vi "Get Angle.vi"(5 "register bus":T3={"Speed"="Speed", "Crank Angle"="Crank Angle", "Cycle Angle"="Cycle Angle", "Crank Count"="Crank Count", "Cycle Count"="Cycle Count", "1.25 MHz Counter"="1.25 MHz Counter", "Crank Rollover"="Crank Rollover", "Cycle Rollover"="Cycle Rollover", "shared settings"={"start"=0.0, "stuck limit"=0.0}} {"shared settings"."start" format="%#.15g"}, 6 "settings.<user name>":T5, 7 "input.<user name>":T2, 11 "state data in":T1) -> (3 "state data out":T1)   [LabVIEW 2013, in "Engine Simulation Toolkit.lvlib" / "Digital Pattern Generation.lvlib"]
uses:
  Digital Pattern Generation.lvlib
  Settings.ctl
  APU/Register Bus.ctl
  APU/Shared Settings.ctl
  Input.ctl
  state data.ctl
  <vilib>/rvi/DataTransferAndStorage/Container/Common/niFpgaContainerExecOnDevCompGetState.vi
  <vilib>/rvi/DataTransferAndStorage/Register/Emulation/niFpgaRegisterEmulationFpgaImpl.vi
  <instcachedir>/0/niFpgaRegisterEmulationFpgaImpl_DCF4BC0110594B98B44A971D60CEEC4D.lvgen/niFpgaRegisterEmulationFpgaImpl_DCF4BC0110594B98B44A971D60CEEC4D_006.vi
  <vilib>/rvi/DataTransferAndStorage/Container/Common/niFpgaContainerGetUniqueNameForEmu.vi
  <vilib>/rvi/DataTransferAndStorage/Container/XNode/niFpgaContainer.xnode
  <vilib>/rvi/DataTransferAndStorage/Register/Emulation/niFpgaRegisterEmulationRefIn.vi
  APU/APU.lvlib
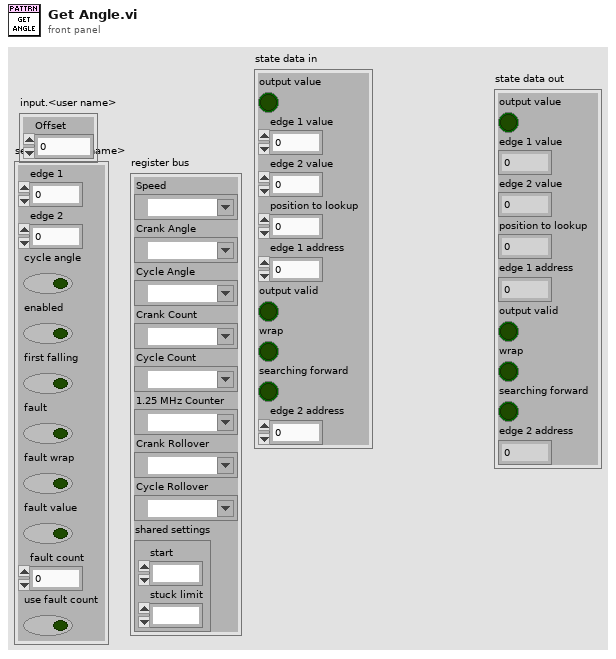
[diagram p1: front panel]
types:
  T1 = typedef "Engine Simulation Toolkit.lvlib/Digital Pattern Generation.lvlib/state data.ctl" = cluster{"output value":bool, "edge 1 value":u16, "edge 2 value":u16, "position to lookup":u16, "edge 1 address":fxp<+,11,11>, "output valid":bool, "wrap":bool, "searching forward":bool, "edge 2 address":fxp<+,11,11>}
  T2 = typedef "Engine Simulation Toolkit.lvlib/Digital Pattern Generation.lvlib/Input.ctl" = cluster{"Offset":i16}
  T3 = typedef "Engine Simulation Toolkit.lvlib/APU.lvlib/Register Bus.ctl" = cluster{"Speed":refnum<k21>, "Crank Angle":refnum<k21>, "Cycle Angle":refnum<k21>, "Crank Count":refnum<k21>, "Cycle Count":refnum<k21>, "1.25 MHz Counter":refnum<k21>, "Crank Rollover":refnum<k21>, "Cycle Rollover":refnum<k21>, "shared settings":T4}
  T4 = typedef "Engine Simulation Toolkit.lvlib/APU.lvlib/Shared Settings.ctl" = cluster{"start":fxp<+,17,17>, "stuck limit":fxp<+,18,18>}
  T5 = typedef "Engine Simulation Toolkit.lvlib/Digital Pattern Generation.lvlib/Settings.ctl" = cluster{"edge 1":u16, "edge 2":u16, "cycle angle":bool, "enabled":bool, "first falling":bool, "fault":bool, "fault wrap":bool, "fault value":bool, "fault count":fxp<+,4,4>, "use fault count":bool}
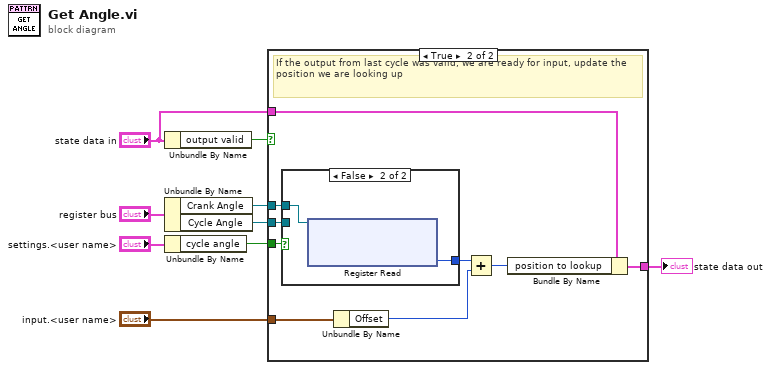
[diagram p0: block diagram]
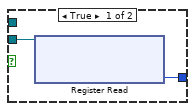
[diagram p3: hidden frame]
diagram:
  n1 = Unbundle By Name("state data in") -> ("output valid"=w1:bool)
  n2 = Unbundle By Name("register bus") -> ("Crank Angle"=w4:refnum<k21>, "Cycle Angle"=w6:refnum<k21>)
  n3 = Unbundle By Name("settings.<user name>") -> ("cycle angle"=w7:bool)
  n4 = case shown="True" w1 {
    tunnel: w7 -> [_ w19]
    tunnel: w6 -> [_ w18]
    tunnel: "state data in" -> [w10 w17]
    tunnel: w4 -> [_ w15]
    tunnel: [w10 w14] -> w2
    tunnel: "input.<user name>" -> [_ w13]
    frame False {
      # "Last cycle the output was not valid, meaning we are still searching, don't touch state data until we are done"
    }
    frame True {
      # "If the output from last cycle was valid, we are ready for input, update the position we are looking up"
      n5 = case shown="False" w19 {
        tunnel: w18 -> [w21 _]
        tunnel: [w20 w22] -> w16
        tunnel: w15 -> [_ w23]
        frame True {
          n6 = xnode ("Register Read")("Register In"=w21) -> ("Data"=w20:u16)  [unwired: 1 out]
        }
        frame False {
          n7 = xnode ("Register Read")("Register In"=w23) -> ("Data"=w22:u16)  [unwired: 1 out]
        }
      }
      n8 = Unbundle By Name(w13) -> ("Offset"=w11:i16)
      n9 = Add(x=w16, y=w11) -> (x+y=w12:u16)
      n10 = Bundle By Name(cluster=w17, "position to lookup"=w12) -> (w14:T1)
    }
  }
  "state data out" <- w2
